vi "myRIO_BRig_RT_dataTrial_Tcycle_Reward.vi"() -> (2 "output_Tcycle_Reward":i32)   [LabVIEW 2014]
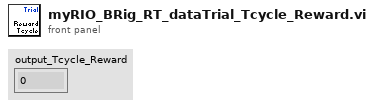
[diagram p1: front panel]
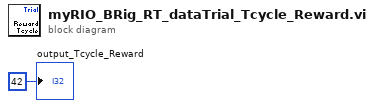
[diagram p0: block diagram]
diagram:
  "output_Tcycle_Reward" <- 42 ("output_iBlock")
